vi "Deadband.vi"(10 "Inputs":dbl[](array[numeric]), 11 "Deadband":dbl) -> (2 "Is Zero?":bool, 3 "Ouptuts":dbl[](array[numeric]))   [LabVIEW 2020]
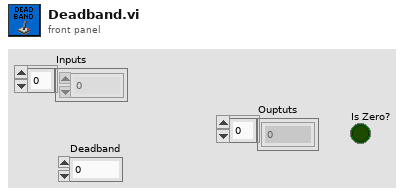
[diagram p1: front panel]
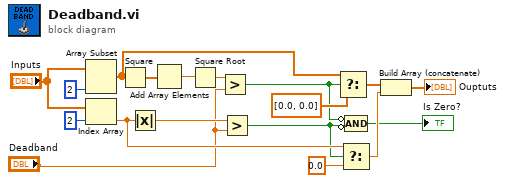
[diagram p0: block diagram]
diagram:
  n1 = Array Subset(array="Inputs", length=2) -> (w12:dbl[])  [unwired: 1 in]
  n2 = Index Array(array="Inputs", index=2) -> (element=w9:dbl)
  n3 = Square(x=w12) -> (x^2=w15:dbl[])
  n4 = Absolute Value(x=w9) -> (abs(x)=w10:dbl)
  n5 = Add Array Elements(numeric array=w15) -> (sum=w14:dbl)
  n6 = Square Root(x=w14) -> (sqrt(x)=w13:dbl)
  n7 = Greater?(x=w13, y="Deadband") -> (0:w4:bool)
  n8 = Greater?(x=w10, y="Deadband") -> (0:w3:bool)
  n9 = Select(t=w12, s=w4, f=dbl[] [0.0, 0.0]) -> (s? t:f=w2:dbl[])
  n10 = Select(t=w9, s=w3, f=0.0) -> (s? t:f=w7:dbl)
  n11 = Compound Arithmetic op=AND(invert w4, invert w3) -> (→"Is Zero?":bool)
  n12 = Build Array (concatenate)(w2, w7) -> (→"Ouptuts":dbl[])
